vi "Coolon.vi"() -> ()   [LabVIEW 2014]
uses:
  ESLSCDLL.dll
panel:
  in  "cool on":bool
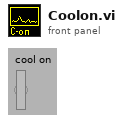
[diagram p1: front panel]
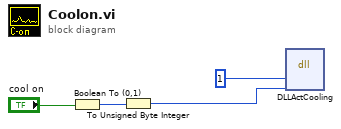
[diagram p0: block diagram]
diagram:
  n1 = Boolean To (0,1)(Boolean="cool on") -> (0, 1=w2:i16)
  n2 = To Unsigned Byte Integer(number=w2) -> (unsigned 8bit integer=w1:u8)
  n3 = dll-call lib="C:/Users/Gerhard/Documents/New64/lv/1cam/board.vis/ESLSCDLL.dll" fn="DLLActCooling"("drv"=u32 1, "on"=w1) -> ()  [unwired: 6 in, 2 out]
